vi "Rhythm.vi"(3 "Sampling rate":dbl, 4 "Segment Length":dbl, 5 "Array":dbl[](array[numeric])) -> (0 "Average Correlation Peak":dbl, 1 "Average Strength":dbl, 2 "Bass Instrumental Onsets":i32)   [LabVIEW 2013]
uses:
  <vilib>/Analysis/4window.llb/Hamming Window (DBL).vi
  <vilib>/Analysis/4window.llb/AllCosWindow (DBL).vi
  <vilib>/measure/macond.llb/Continuous Waveform Convolution for 1 Chan.vi
  <vilib>/Analysis/NI_AAL_SigProc.lvlib
  <vilib>/Analysis/NI_AALPro.lvlib
  <vilib>/measure/NI_MAPro.lvlib
panel:
  out "sub-band":waveform(dbl)(graph)
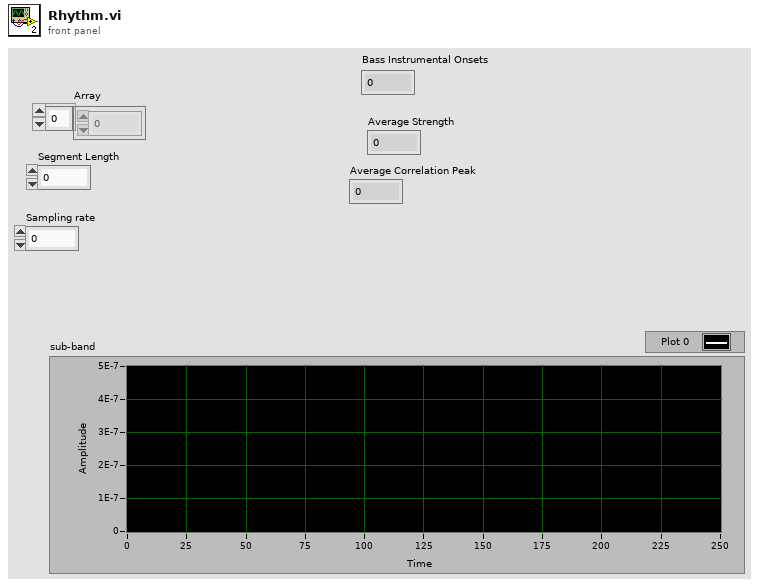
[diagram p1: front panel]
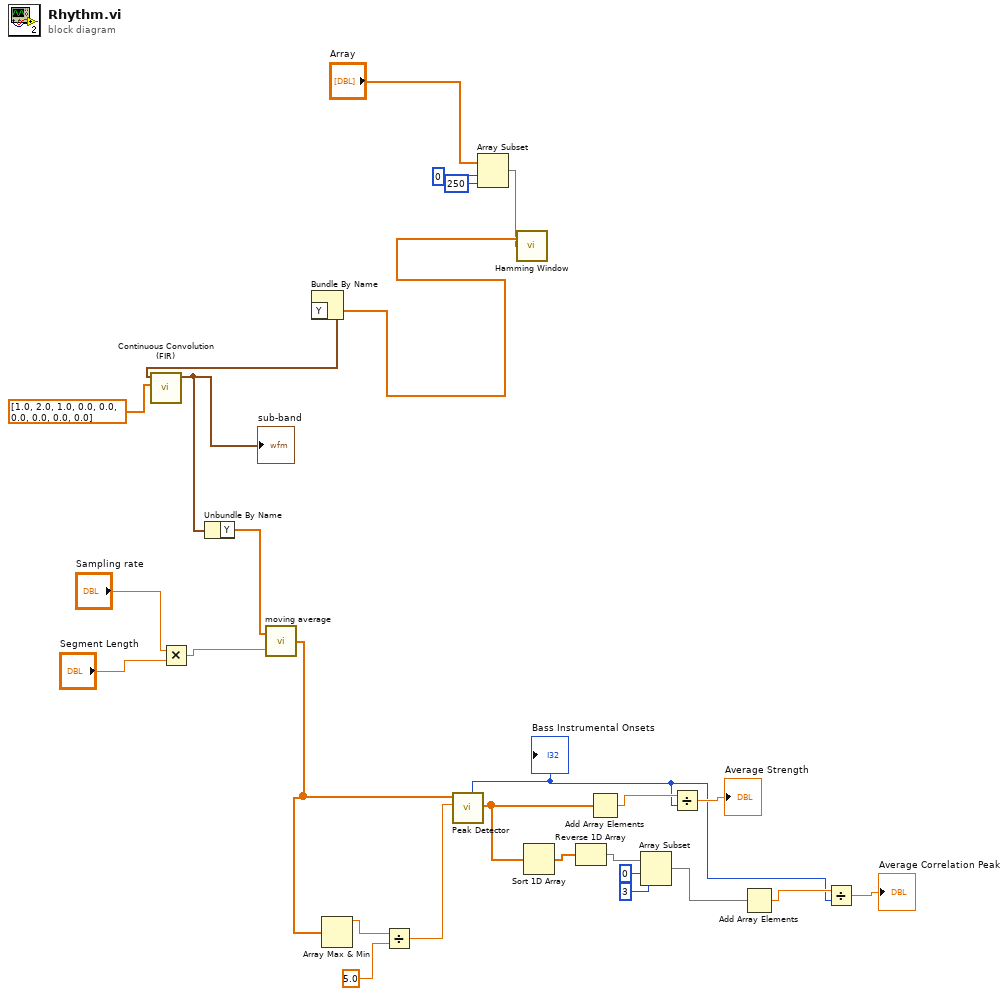
[diagram p0: block diagram]
diagram:
  n1 = Multiply(x="Sampling rate", y="Segment Length") -> (x*y=w1:dbl)
  n2 = Array Subset(array="Array", index=0, length=250) -> (w8:dbl[])
  n3 = call-poly <vilib>:"Hamming Window.vi"("X"=w8) -> ("Windowed X"=w10:dbl[])  [unwired: 1 out]
  n4 = Bundle By Name("Y"=w10) -> (w11:waveform(dbl))  [unwired: 1 in]
  n5 = call-poly <vilib>:"Continuous Convolution (FIR).vi"("kernel"=dbl[] [1.0, 2.0, 1.0, 0.0, 0.0, 0.0, 0.0, 0.0, 0.0] ("kernel 2"), "signal in"=w11) -> ("signal out"=w13:waveform(dbl))  [unwired: 8 in, 1 out]
  "sub-band" <- w13
  n6 = Unbundle By Name(w13) -> ("Y"=w5:dbl[])
  n7 = call "moving average.vi"("length"=w1, "raw array"=w5) -> ("averaged array"=w4:dbl[])
  n8 = Array Max & Min(array=w4) -> (max value=w27:dbl)  [unwired: 3 out]
  n9 = Divide(x=w27, y=5.0) -> (x/y=w25:dbl)
  n10 = call <vilib>:"Peak Detector.vi"("threshold"=w25, "X"=w4) -> ("Amplitudes"=w15:dbl[], "# found"=w14:i32)  [unwired: 5 in, 3 out]
  "Bass Instrumental Onsets" <- w14
  n11 = Sort 1D Array(array=w15) -> (sorted array=w22:dbl[])
  n12 = Reverse 1D Array(array=w22) -> (reversed array=w21:dbl[])
  n13 = Add Array Elements(numeric array=w15) -> (sum=w24:dbl)
  n14 = Array Subset(array=w21, index=0, length=3) -> (w16:dbl[])
  n15 = Divide(x=w24, y=w14) -> (x/y=→"Average Strength":dbl)
  n16 = Add Array Elements(numeric array=w16) -> (sum=w18:dbl)
  n17 = Divide(x=w18, y=w14) -> (x/y=→"Average Correlation Peak":dbl)
